vi "Path配置.vi"() -> (2 "确定":bool)   [LabVIEW 2020]
uses:
  Global.vi
  <vilib>/Utility/file.llb/Write Delimited Spreadsheet (string).vi
panel:
  in  "Path":path
  in  "Path":string="D:\\MES"
  in  "取消":bool
  in  "确定":bool
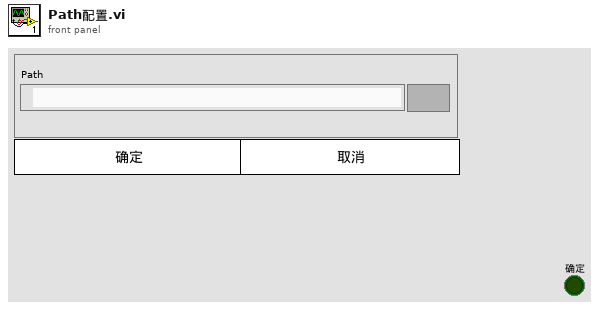
[diagram p1: front panel]
types:
  T1 = cluster{"Server":string, "audit_mode":string, "tsid":string, "model":string, "product":string, "test_station":string, "station_id":string, "test_station_name":string, "Webservice":string}
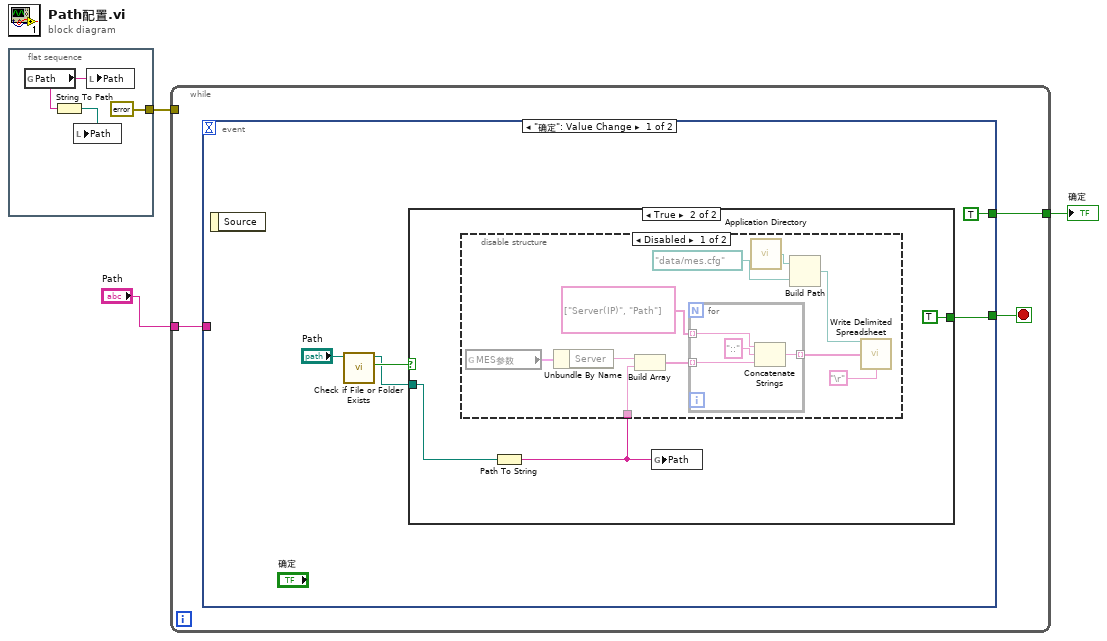
[diagram p0: block diagram]
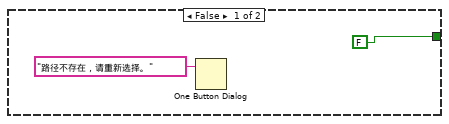
[diagram p2: hidden frame]
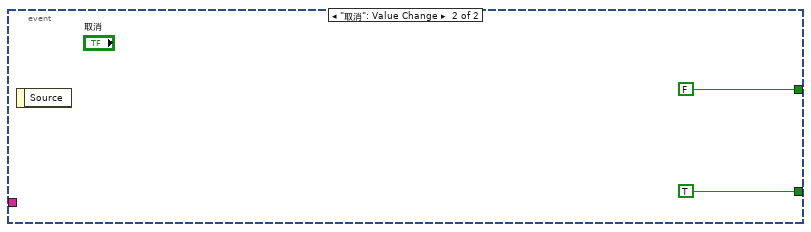
[diagram p4: hidden frame]
diagram:
  n1 = flat-sequence {
    tunnel: [errorcluster {"status"=FALSE, "code"=0, "source"=""} ("错误常量")] -> w2
    frame #0 {
      n2 = global read "Global.vi" "Path"() -> (w5:string)
      n3 = String To Path(string=w5) -> (path=w4:path)
      n4 = local write "Path"(w4) -> ()
      n5 = local write "Path"(w5) -> ()
    }
  }
  n6 = while {
    tunnel: [w8] -> w3
    tunnel: w2 -> [_]
    tunnel: "Path" -> [w7]
    stop <- w9 stop-if-true
    n7 = event shown="[0] \"确定\": Value Change" {
      selector: _ -> [_ _]
      dyn-events: _ -> [_ _]
      timeout: _ -> [_ _]
      tunnel: [w10 TRUE] -> w9
      tunnel: [TRUE FALSE] -> w8
      tunnel: w7 -> [_ _]
      event "确定": Value Change {
        n8 = event-data() -> ()  [unwired: 1 in, 1 out]
        n9 = call <vilib>:"Check if File or Folder Exists.vi"("path"="Path") -> ("file or folder exists?"=w12:bool, "dup path"=w11:path)  [unwired: 8 in, 1 out]
        n10 = case shown="True" w12 {
          tunnel: w11 -> [_ w19]
          tunnel: [FALSE TRUE] -> w10
          frame False {
            n11 = One Button Dialog(message="路径不存在，请重新选择。") -> ()  [unwired: 1 in, 1 out]
          }
          frame True {
            n12 = Path To String(path=w19) -> (string=w18:string)
            n13 = disable-structure shown="Disabled" {
              disable-tunnel: w18 -> [w20 _]
              frame Disabled {
                n14 = global read "Global.vi" "MES参数"() -> (w22:T1)
                n15 = Unbundle By Name(w22) -> ("Server"=w21:string)
                n16 = Build Array(w21, w20) -> (w25:string[])
                n17 = for {
                  tunnel: string[] ["Server(IP)", "Path"] ("转置的数组") -> [w33] mode=indexing
                  tunnel: w25 -> [w31] mode=indexing
                  tunnel: [w30] -> w24 mode=indexing
                  n18 = Concatenate Strings(w33, "::" ("String"), w31) -> (w30:string)
                }
                n19 = call <vilib>:"Application Directory.vi"() -> ("Application Directory"=w28:path)
                n20 = Build Path(base path=w28, name or relative path=path "data/mes.cfg") -> (appended path=w27:path)
                n21 = call-poly <vilib>:"Write Delimited Spreadsheet.vi"("file path (dialog if empty)"=w27, "1D data"=w24, "delimiter (\\t)"="\r") -> ()  [unwired: 11 in, 2 out]
              }
              frame Enabled {
              }
            }
            n22 = global write "Global.vi" "Path"(w18) -> ()
          }
        }
      }
      event "取消": Value Change {
        n23 = event-data() -> ()  [unwired: 1 in, 1 out]
      }
    }
  }
  "确定" <- w3
